vi "APC_PC_UI_Main.vi"() -> ()   [LabVIEW 2020]
uses:
  controls/APC_ControlSettings.ctl
  controls/APC_PIDcontrolSettings.ctl
  controls/APC_SavingFile.ctl
  controls/APC_ErrorCluster.ctl
panel:
  in  "Tab Control 2":enum32{"Main view", "Aux", "Test"}(tab)
  out "PYTHON \n(effective)":bool
  in  "Python in \ncommand":bool
  out "Cylinder pressure state":u32[][](array[colorbox])
  out "CA50 [CADATDC]":dbl format="%#.2f"
  in  "CA50 ref [CADBTDC]":dbl
  out "SA [CADBTDC]":dbl format="%#_2f"
  in  "Listbox":i32(listbox)
  in  "Override system view references":bool=TRUE
  out "NG flow [kg/h]":dbl format="%#.5f"
  in  "Cycles":u16=1 min=1 max=1000
  out "Saving info":string
  in  "Transfer CRIO9056":bool
  in  "Transfer CRIO9049":bool
  in  "Test notes auto erase":string="(auto-erased note)\n"
  in  "Pre-trigger":bool
  in  "Record Button":bool
  in  "Test code":string
  in  "Test ID":u32=1
  in  "Test notes":string
  in  "CO2ref":dbl
  in  "O2ref":dbl
  in  "Pref":dbl
  out "CO2 [%]":dbl format="%#.2f"
  in  "Force motoring":bool
  in  "Force idling":bool
  out "Max p [bar]":dbl[](array[numeric]) format="%#.2g"
  out "IMEP s":dbl[](array[numeric]) format="%#.2f"
  out "IMEP [bar]":dbl[](array[numeric]) format="%#.2f"
  in  "l ref":dbl format="%#.4f"
  out "l":dbl format="%#_2f"
  in  "NG flow ref":dbl format="%#.2f"
  in  "PFI enable switch":bool=TRUE
  in  "DI duration [ms]":dbl=1.0
  in  "DI advance [CADBTDC]":dbl=160.0
  in  "DI enable switch":bool=TRUE
  in  "Spark Advance [CADBTDC]":dbl
  in  "IGN enable switch":bool=TRUE
  in  "Speed setting selector":bool
  in  "Low speed setting":dbl=900.0
  in  "High speed setting":dbl=1800.0
  in  "EMERGENCY STOP":bool
  out "Warning":bool
  in  "Clear warning":bool
  out "n [rpm]":dbl
  out "Gauge":dbl(knob)=1148.34130859375 scale=0.0..2000.0
  out "Stand-by":bool
  out "Motoring":bool
  out "Firing":bool
  out "Idling":bool
  out "Emergency":bool
  out "System pressure [bar]":dbl format="%#.2f"
  out "NOx [ppm]":dbl format="%#.1f"
  out "O2 [%]":dbl format="%#.2f"
  out "Waveform Graph":dbl[][](graph)
  in  "PFI control selector":enum32{"PFI NG flow", "CL PFI  lambda"}(radio)
  in  "CL SA CA50":bool
  in  "knock limiter":bool
  out "Texh":bool
  out "control system":bool
  out "NG feed":bool
  out "NG control":bool
  out "membrane control":bool
  out "dyno control":bool
  out "Intake vent":bool
  out "NOx contamination":bool
  out "Ar feed":bool
  out "O2 feed":bool
  out "oil pressure":bool
  out "engine cooling":bool
  out "pexh":bool
  out "oil temperature":bool
  out "exhaust vent":bool
  out "cross vent":bool
  out "O2 control":bool
  out "system pressure":bool
  out "System error lookup":u32[][](array[colorbox])
  in  "Requested mode":i8(slide) scale=-1.0..3.0
  out "9056_PCnotResponding":bool
  out "9056_9049notResponding":bool
  out "9056_MTRnotResponding":bool
  out "Iteration Count":i32
  out "SystemState":dbl
  in  "ETP resync":bool
  in  "toggle \nTDC":bool
  in  "Activate\ncylinder":bool[](array[boolean])=[TRUE, TRUE, TRUE, TRUE, TRUE, TRUE]
  out "Emergency Stop Boolean":bool
  out "After 1st box":i8
  out "After 2nd box":i8
  out "After 3rd box":i8
  out "After 4th box":i8
  # "Raster 1"
  # "Raster 2"
  # "Raster 3"
  # "Raster 4"
  # "Raster 5"
  # "monarch APC v0.1"
  # "late comb"
  # "cyclic var"
  # "misfire 1"
  # "misfire 2"
  # "misfire 3"
  # "knock"
  # "Pmax"
  # "Knock limiter disabled"
  # "CA50 Control disabled"
  # "MC lambda control disabled"
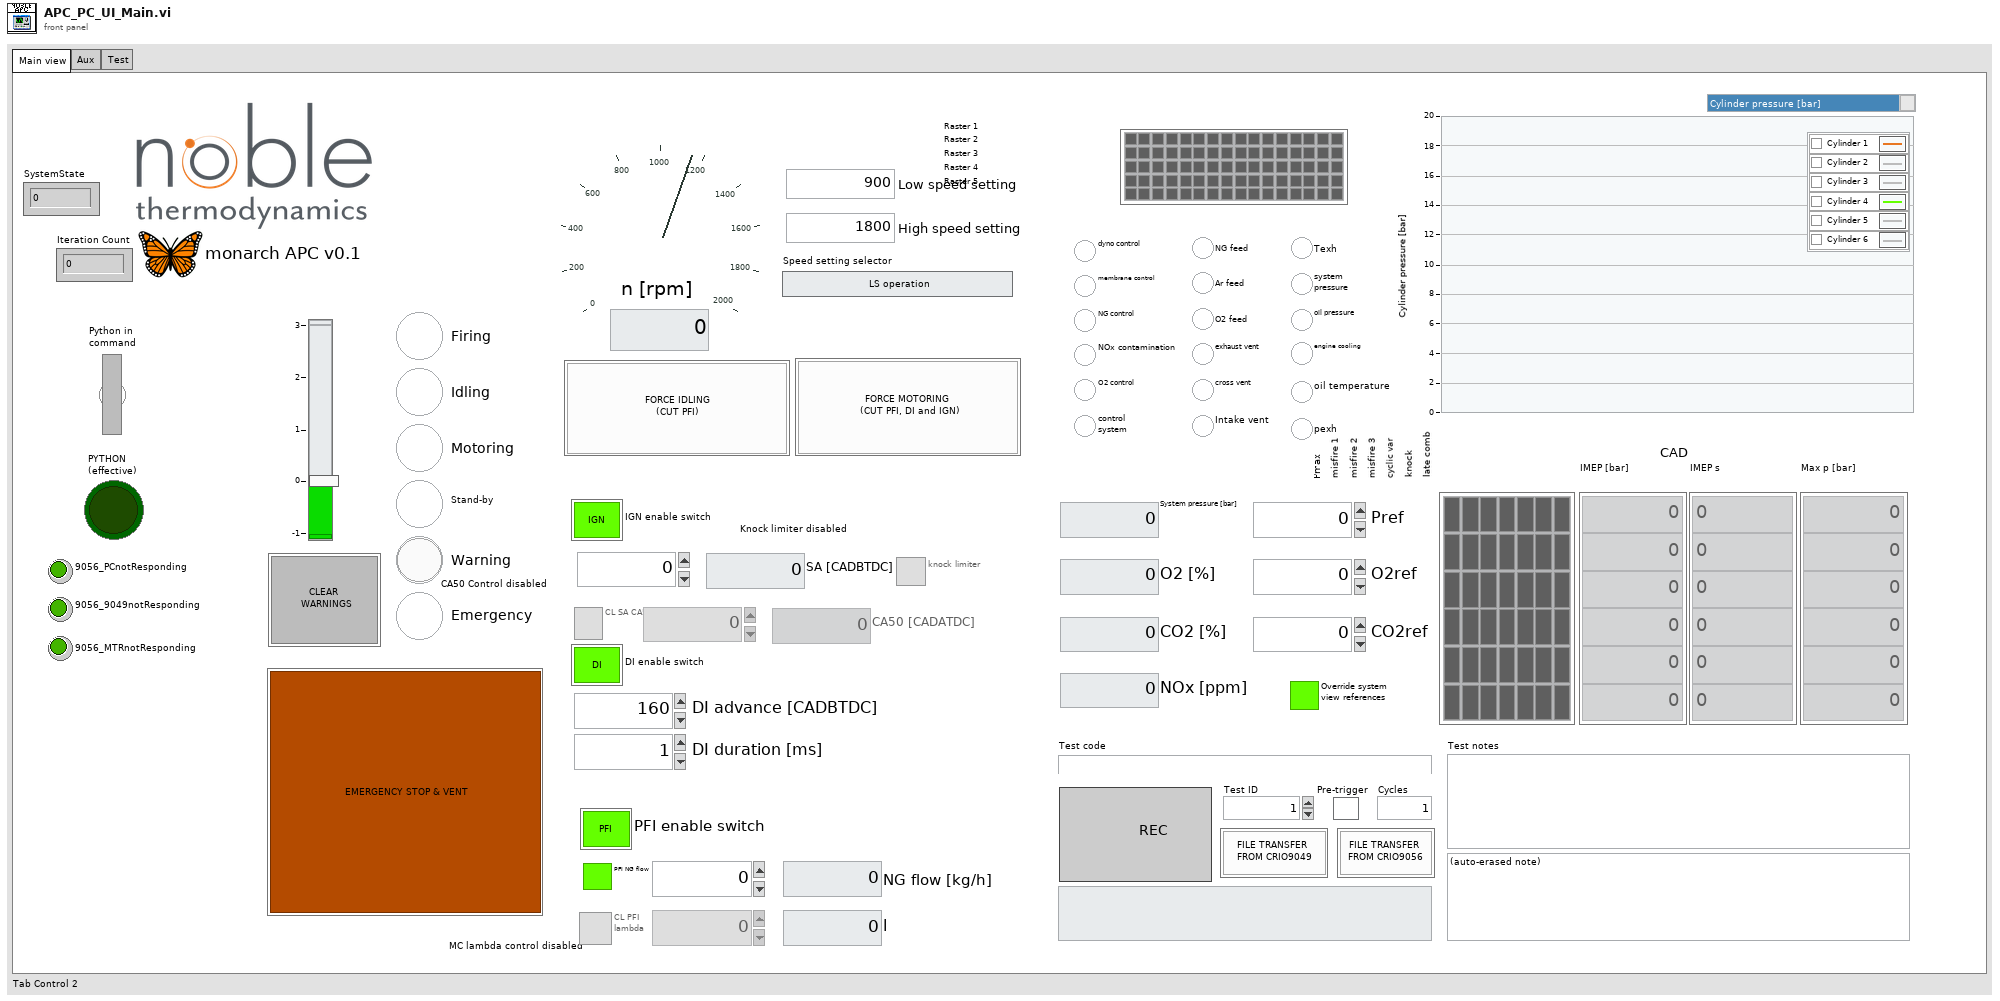
[diagram p1: front panel]
types:
  T1 = enum8{"Enabled", "Disabled", "Disabled and Grayed Out"}
  T2 = typedef "APC_ControlSettings.ctl" = cluster{"Spark advance [CADBTDC]":dbl, "Pref":dbl, "O2ref":dbl, "DI advance [CADBTDC]":dbl, "DI duration [ms] ":dbl, "CO2ref":dbl, "PFI duration [ms]":dbl, "IMEP ref":dbl, "Speed ref":dbl, "IGN enable":bool, "DI enable":bool, "CL PFI\n lambda":bool, "CL PFI\nIMEP":bool, "Activate\ncylinder":bool[], "Force idling":bool, "Force motoring":bool, "ETP resync":bool, "Requested mode":i8, "Clear Sync Errors":bool, "toggle TDC":bool, "l ref":dbl, "PID control references":T3, "CA50setpoint [CADATDC]":dbl, "CA50 control":bool, "Knock control":bool, "CLEAR EMERGENCY STOP":bool, "EMERGENCY STOP":bool}
  T3 = typedef "APC_PIDcontrolSettings.ctl" = cluster{"NG":bool, "Ar":bool, "O2":bool, "Intake vent":bool, "Cross vent":bool, "Exhaust vent":bool, "NG control mode":u8, "NG-FC-001-REF":dbl, "WF-OA-002-REF":dbl, "IMEP-REF":dbl, "Nm-REF":dbl, "Ar control mode":u8, "AR-PC-002-REF":dbl, "WF-PT-004-REF":dbl, "O2 control mode":u8, "O2-FC-001-REF":dbl, "WF-OA-001-REF":dbl, "Tcoolant control  mode":u8, "EC-FC-001-REF":dbl, "EC-TT-001-REF":dbl, "Texh control mode":u8, "SW-FC-004-REF":dbl, "SW-FT-002-REF":dbl, "WF-TT-004-REF":dbl, "Toil control mode":u8, "SW-FC-009-REF":dbl, "SW-FT-004-REF":dbl, "EO-TT-001-REF":dbl, "AIC201_CO2_ConcTarget":dbl, "O2_FF_NG":bool, "Dyno control mode":u8, "Membrane control mode":u8, "AR-FT-001-REF":dbl, "MTR modbus floats":sgl[], "MTR modbus u16":u16[], "MTR HB":bool, "PC_HB":bool, "EMERGENCY STOP":bool}
  T4 = typedef "APC_ErrorCluster.ctl" = cluster{"AI and system state":u32[][], "Cylinder pressure state":u32[][], "EMERGENCY STOP":bool}
  T5 = typedef "APC_VisualizationCluster_v2.ctl" = cluster{"AR-FT-001":dbl, "AR-PT-001":dbl, "AR-TT-001":dbl, "AT103_CO2Conc":dbl, "AT201_CO2Conc":dbl, "C101_CompSpeed_rpm":dbl, "CO2 [%]":dbl, "EC-FC-001":dbl, "EC-TT-001":dbl, "EC-TT-002":dbl, "PC-TT-001":dbl, "PC-TT-002":dbl, "PC-TT-003":dbl, "PC-TT-004":dbl, "PC-TT-005":dbl, "PC-TT-006":dbl, "EO-PT-001":dbl, "EO-TT-001":dbl, "EO-TT-002":dbl, "FT301_Flow_kgh":dbl, "FV301_VlvPos_pc_fb":dbl, "IMEPn1":dbl, "IMEPn2":dbl, "IMEPn3":dbl, "IMEPn4":dbl, "IMEPn5":dbl, "IMEPn6":dbl, "IMEPstd1":dbl, "IMEPstd2":dbl, "IMEPstd3":dbl, "IMEPstd4":dbl, "IMEPstd5":dbl, "IMEPstd6":dbl, "NG-FC-001":dbl, "NG-FT-001":dbl, "NG-PT-001":dbl, "NG-TT-001":dbl, "NGDI-FT-001":dbl, "NGDI-PT-001":dbl, "NGDI-TT-001":dbl, "WF-OA-002-NOx":dbl, "TORQUE":dbl, "WF-OA-002-O2corr":dbl, "O2-FC-001":dbl, "O2-PT-001":dbl, "O2-TT-001":dbl, "PT103_Pressure_kPa":dbl, "PT104_Pressure_kPa":dbl, "PT106_Pressure_kPa":dbl, "PT300_Pressure_kPa":dbl, "PV103_VlvPos_pc_fb":dbl, "PV300_VlvPos_pc_fb":dbl, "MaxPcyl1":dbl, "MaxPcyl2":dbl, "MaxPcyl3":dbl, "MaxPcyl4":dbl, "MaxPcyl5":dbl, "MaxPcyl6":dbl, "SW-FC-004":dbl, "SW-FC-009":dbl, "SW-FT-001":dbl, "SW-FT-002":dbl, "SW-FT-003":dbl, "SW-FT-004":dbl, "SW-TT-001":dbl, "SW-TT-002":dbl, "SW-TT-003":dbl, "SW-TT-004":dbl, "SW-TT-005":dbl, "SW-TT-006":dbl, "SW-TT-007":dbl, "SW-TT-008":dbl, "WF-OA-001":dbl, "WF-OA-002":dbl, "WF-PT-001":dbl, "WF-PT-004":dbl, "WF-PT-005avg":dbl, "WF-PT-014":dbl, "WF-PT-015":dbl, "WF-PT-016":dbl, "WF-TT-001":dbl, "WF-TT-002":dbl, "WF-TT-003":dbl, "WF-TT-004":dbl, "WF-TT-007":dbl, "EngineSpeed_rpm":dbl, "SystemState":dbl, "CylPresWarnings":dbl, "CylPresErrors":dbl, "MAPO1":dbl, "MAPO2":dbl, "MAPO3":dbl, "MAPO4":dbl, "MAPO5":dbl, "MAPO6":dbl, "CA50_1":dbl, "CA50_2":dbl, "CA50_3":dbl, "CA50_4":dbl, "CA50_5":dbl, "CA50_6":dbl, "SparkTiming":dbl, "SW-TT-009":dbl, "NG-FV-001":dbl, "O2-PV-004":dbl, "AR-PV-004":dbl, "WF-FC-001":dbl, "WF-FC-002":dbl, "WF-FC-003":dbl, "WF-PT-012avg":dbl}
  T6 = typedef "APC_SavingFile.ctl" = cluster{"TEST CODE":string, "ID":u32, "FLUSH and SAVE BUFFER":bool, "REC BUFFER":bool, "Test Notes":string, "Cycles":u16}
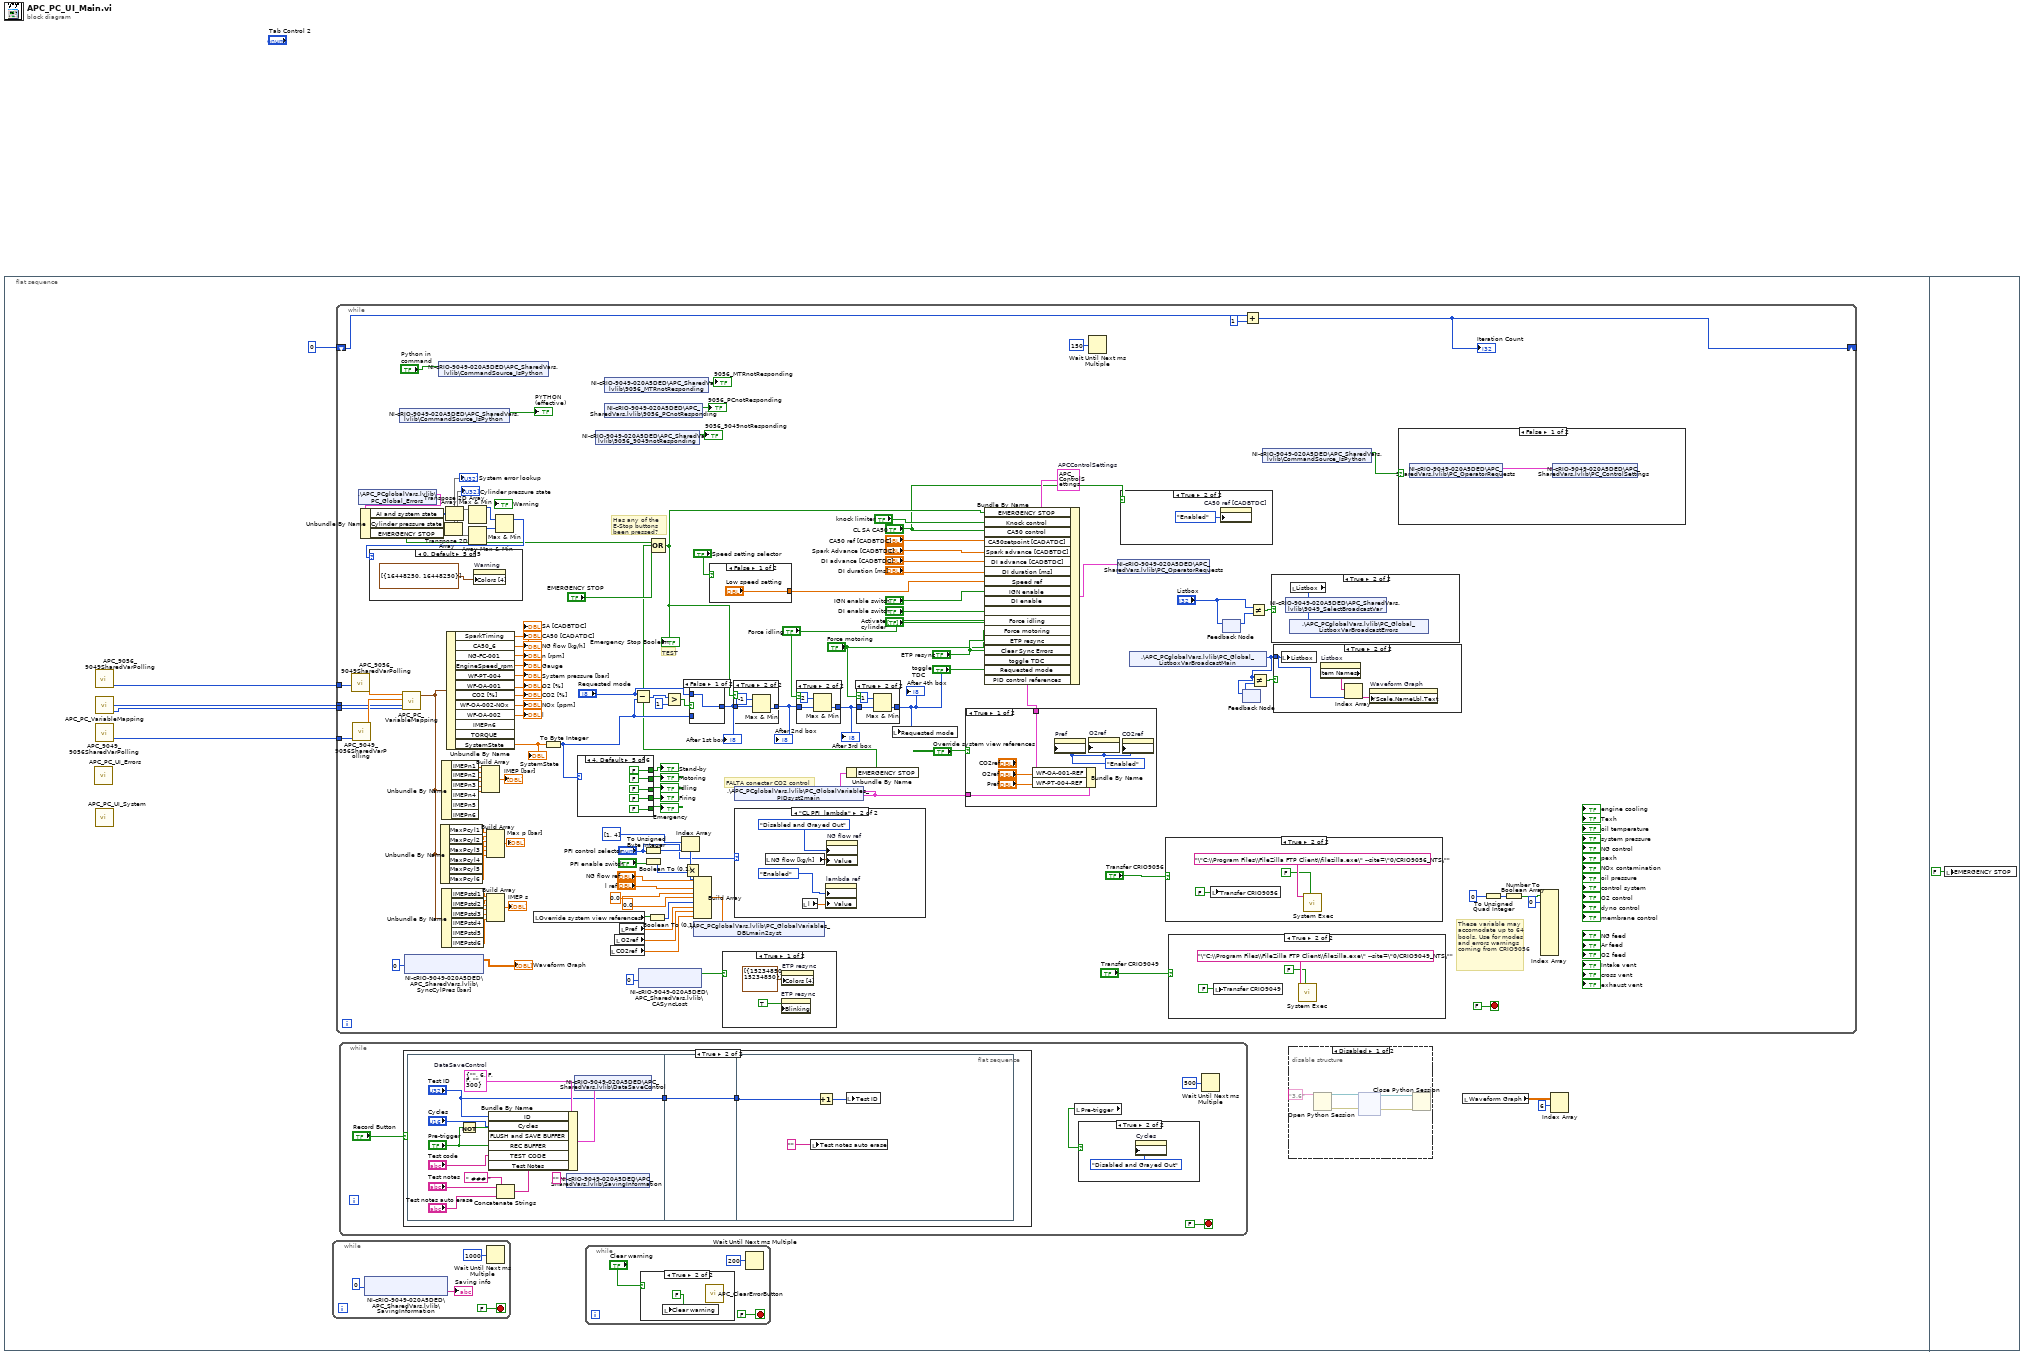
[diagram p0: block diagram]
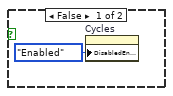
[diagram p3: hidden frame]
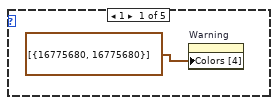
[diagram p7: hidden frame]
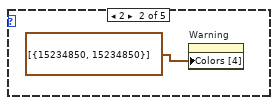
[diagram p8: hidden frame]
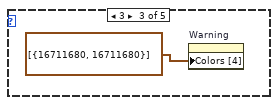
[diagram p9: hidden frame]
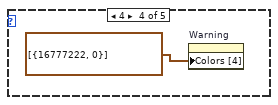
[diagram p10: hidden frame]
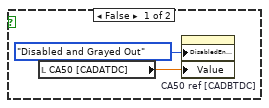
[diagram p11: hidden frame]
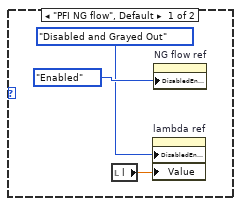
[diagram p12: hidden frame]
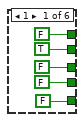
[diagram p16: hidden frame]
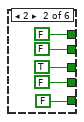
[diagram p17: hidden frame]
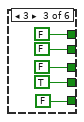
[diagram p18: hidden frame]
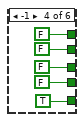
[diagram p19: hidden frame]
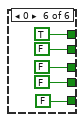
[diagram p20: hidden frame]
diagram:
  n1 = flat-sequence {
    frame #0 {
      n2 = call "APC_PC_UI_Errors.vi"() -> ()  [unwired: 12 in]
      n3 = call "APC_9056_9049SharedVarPolling.vi"() -> ("Number of signals (out)"=w5:i32)  [unwired: 1 in, 1 out]
      n4 = call "APC_PC_UI_System.vi"() -> ()  [unwired: 12 in]
      n5 = call "APC_PC_VariableMapping.vi"() -> ("Index 9056"=w6:i32[], "Index 9049"=w7:i32[])  [unwired: 4 in, 1 out]
      n6 = call "APC_9049_9056SharedVarPolling.vi"() -> ("Number of signals (out)"=w4:i32)  [unwired: 1 in, 3 out]
      n7 = while {
        stop <- FALSE stop-if-true
        n8 = shared-variable "NI-cRIO-9049-020A5DED\\APC_SharedVars.lvlib\\SavingInformation"(0 ("ms timeout (0)")) -> (→"Saving info":string)  [unwired: 1 in, 2 out]
        n9 = Wait Until Next ms Multiple(millisecond multiple=u32 1000) -> ()  [unwired: 1 out]
      }
      n10 = while {
        tunnel: w7 -> [w163]
        tunnel: w6 -> [w162]
        tunnel: w5 -> [w161]
        tunnel: w4 -> [w160]
        shift-right: [w53] -> _
        shift-left: 0 -> [w55]
        stop <- FALSE stop-if-true
        w157 = T2 {"Spark advance [CADBTDC]"=0.0, "Pref"=0.0, "O2ref"=0.0, "DI advance [CADBTDC]"=0.0, "DI duration [ms] "=0.0, "CO2ref"=0.0, "PFI duration [ms]"=0.0, "IMEP ref"=0.0, "Speed ref"=1800.0, "IGN enable"=TRUE, "DI enable"=TRUE, "CL PFI\n lambda"=FALSE, "CL PFI\nIMEP"=FALSE, "Activate\ncylinder"=[FALSE, FALSE, FALSE, FALSE, FALSE, FALSE], "Force idling"=FALSE, "Force motoring"=FALSE, "ETP resync"=FALSE, "Requested mode"=0, "Clear Sync Errors"=FALSE, "toggle TDC"=FALSE, "l ref"=0.0, "PID control references"={"NG"=FALSE, "Ar"=FALSE, "O2"=FALSE, "Intake vent"=FALSE, "Cross vent"=FALSE, "Exhaust vent"=FALSE, "NG control mode"=0, "NG-FC-001-REF"=0.0, "WF-OA-002-REF"=0.0, "IMEP-REF"=0.0, "Nm-REF"=0.0, "Ar control mode"=0, "AR-PC-002-REF"=0.0, "WF-PT-004-REF"=0.0, "O2 control mode"=0, "O2-FC-001-REF"=0.0, "WF-OA-001-REF"=0.0, "Tcoolant control  mode"=0, "EC-FC-001-REF"=0.0, "EC-TT-001-REF"=0.0, "Texh control mode"=0, "SW-FC-004-REF"=0.0, "SW-FT-002-REF"=0.0, "WF-TT-004-REF"=0.0, "Toil control mode"=0, "SW-FC-009-REF"=0.0, "SW-FT-004-REF"=0.0, "EO-TT-001-REF"=0.0, "AIC201_CO2_ConcTarget"=0.0, "O2_FF_NG"=FALSE, "Dyno control mode"=0, "Membrane control mode"=0, "AR-FT-001-REF"=0.0, "MTR modbus floats"=[0.0, 0.0, 0.0, 0.0, 0.0, 0.0, 0.0, 0.0, 0.0, 0.0, 0.0, 0.0, 0.0, 0.0, 0.0, 0.0, 0.0, 0.0, 0.0], "MTR modbus u16"=[0, 0, 0, 0, 0, 0, 0], "MTR HB"=FALSE, "PC_HB"=FALSE, "EMERGENCY STOP"=FALSE}, "CA50setpoint [CADATDC]"=0.0, "CA50 control"=TRUE, "Knock control"=FALSE, "CLEAR EMERGENCY STOP"=FALSE, "EMERGENCY STOP"=FALSE}  # APCControlSettings
        # "TEST"
        # "Has any of the E-Stop buttons been pressed?"
        # "These variable may accomodate up to 64 bools. Use for modes and errors warnings coming from CRIO9056"
        # "FALTA conectar CO2 control"
        n11 = call "APC_9056_9049SharedVarPolling.vi"("Number of signals"=w161) -> ("9049_CycleAveragedVariables"=w165:dbl[])  [unwired: 1 out]
        n12 = call "APC_9049_9056SharedVarPolling.vi"("Number of signals"=w160) -> ("9056 IO"=w164:dbl[])  [unwired: 3 out]
        n13 = shared-variable ".\\APC_PCglobalVars.lvlib\\PC_Global_Errors"() -> (w74:T4)  [unwired: 1 in, 1 out]
        n14 = Unbundle By Name(w74) -> ("AI and system state"=w72:u32[][], "Cylinder pressure state"=w73:u32[][], "EMERGENCY STOP"=w66:bool)
        n15 = shared-variable "NI-cRIO-9049-020A5DED\\APC_SharedVars.lvlib\\CommandSource_IsPython"() -> (→"PYTHON \n(effective)":bool)  [unwired: 1 in, 1 out]
        n16 = call "APC_PC_VariableMapping.vi"("Index of array for 9056"=w162, "Index of array for 9049"=w163, "9056 IO"=w164, "9049_CycleAveragedVariables"=w165) -> ("Output cluster"=w61:T5)  [unwired: 2 out]
        n17 = shared-variable "NI-cRIO-9049-020A5DED\\APC_SharedVars.lvlib\\SyncCylPres [bar]"(0 ("ms timeout (0)")) -> (→"Waveform Graph":dbl[][])  [unwired: 1 in, 2 out]
        n18 = shared-variable "NI-cRIO-9049-020A5DED\\APC_SharedVars.lvlib\\CommandSource_IsPython"("Python in \ncommand") -> ()  [unwired: 1 in, 1 out]
        n19 = Unbundle By Name(w61) -> ("MaxPcyl1"=w138:dbl, "MaxPcyl2"=w139:dbl, "MaxPcyl3"=w134:dbl, "MaxPcyl4"=w135:dbl, "MaxPcyl5"=w136:dbl, "MaxPcyl6"=w137:dbl)
        n20 = Unbundle By Name(w61) -> ("IMEPn1"=w145:dbl, "IMEPn2"=w146:dbl, "IMEPn3"=w141:dbl, "IMEPn4"=w142:dbl, "IMEPn5"=w143:dbl, "IMEPn6"=w144:dbl)
        n21 = Unbundle By Name(w61) -> ("IMEPstd1"=w131:dbl, "IMEPstd2"=w132:dbl, "IMEPstd3"=w127:dbl, "IMEPstd4"=w128:dbl, "IMEPstd5"=w129:dbl, "IMEPstd6"=w130:dbl)
        n22 = Transpose 2D Array(2D array=w73) -> (transposed array=w71:u32[][])
        "Cylinder pressure state" <- w71
        n23 = Transpose 2D Array(2D array=w72) -> (transposed array=w70:u32[][])
        "System error lookup" <- w70
        n24 = Unbundle By Name(w61) -> ("SparkTiming"=→"SA [CADBTDC]":dbl, "CA50_6"=→"CA50 [CADATDC]":dbl, "NG-FC-001"=→"NG flow [kg/h]":dbl, "EngineSpeed_rpm"=→"Gauge" →"n [rpm]":dbl, "WF-PT-004"=→"System pressure [bar]":dbl, "WF-OA-001"=→"O2 [%]":dbl, "CO2 [%]"=→"CO2 [%]":dbl, "WF-OA-002-NOx"=→"NOx [ppm]":dbl, "WF-OA-002"=→"l":dbl, "SystemState"=w91:dbl)  [unwired: 2 out]
        "SystemState" <- w91
        n25 = Array Max & Min(array=w71) -> (max value=w69:u32)  [unwired: 3 out]
        n26 = Array Max & Min(array=w70) -> (max value=w68:u32)  [unwired: 3 out]
        n27 = Build Array(w145, w146, w141, w142, w143, w144) -> (→"IMEP [bar]":dbl[])
        n28 = Build Array(w138, w139, w134, w135, w136, w137) -> (→"Max p [bar]":dbl[])
        n29 = Build Array(w131, w132, w127, w128, w129, w130) -> (→"IMEP s":dbl[])
        n30 = Max & Min(x=w69, y=w68) -> (max(x,y)=w67:u32)  [unwired: 1 out]
        n31 = case shown="0, Default" w67 {
          frame 1 {
            n32 = property on="Warning" class="Bool (strict)"("Colors [4]"=cluster{u32, u32}[] [{16775680, 16775680}]) -> ()  [unwired: 2 in, 2 out]
          }
          frame 2 {
            n33 = property on="Warning" class="Bool (strict)"("Colors [4]"=cluster{u32, u32}[] [{15234850, 15234850}]) -> ()  [unwired: 2 in, 2 out]
          }
          frame 3 {
            n34 = property on="Warning" class="Bool (strict)"("Colors [4]"=cluster{u32, u32}[] [{16711680, 16711680}]) -> ()  [unwired: 2 in, 2 out]
          }
          frame 4 {
            n35 = property on="Warning" class="Bool (strict)"("Colors [4]"=cluster{u32, u32}[] [{16777222, 0}]) -> ()  [unwired: 2 in, 2 out]
          }
          frame 0, Default {
            n36 = property on="Warning" class="Bool (strict)"("Colors [4]"=cluster{u32, u32}[] [{16448250, 16448250}]) -> ()  [unwired: 2 in, 2 out]
          }
        }
        n37 = local read "Override system view references"() -> (w105:bool)
        n38 = To Byte Integer(number=w91) -> (8bit integer=w90:i8)
        n39 = case shown="4, Default" w90 {
          tunnel: [FALSE ("Stand-by") FALSE ("Stand-by") FALSE ("Stand-by") FALSE ("Stand-by") FALSE ("Stand-by") TRUE ("Stand-by")] -> w89
          tunnel: [TRUE ("Stand-by") FALSE ("Stand-by") FALSE ("Stand-by") FALSE ("Stand-by") FALSE ("Stand-by") FALSE ("Stand-by")] -> w87
          tunnel: [FALSE ("Stand-by") FALSE ("Stand-by") FALSE ("Stand-by") TRUE ("Stand-by") FALSE ("Stand-by") FALSE ("Stand-by")] -> w88
          tunnel: [FALSE ("Stand-by") TRUE ("Stand-by") FALSE ("Stand-by") FALSE ("Stand-by") FALSE ("Stand-by") FALSE ("Stand-by")] -> w86
          tunnel: [FALSE ("Stand-by") FALSE ("Stand-by") TRUE ("Stand-by") FALSE ("Stand-by") FALSE ("Stand-by") FALSE ("Stand-by")] -> w85
          frame 1 {
          }
          frame 2 {
          }
          frame 3 {
          }
          frame -1 {
          }
          frame 4, Default {
          }
          frame 0 {
          }
        }
        "Stand-by" <- w89
        "Motoring" <- w87
        "Firing" <- w85
        "Idling" <- w86
        "Emergency" <- w88
        n40 = shared-variable "NI-cRIO-9049-020A5DED\\APC_SharedVars.lvlib\\9056_9049notResponding"() -> (→"9056_9049notResponding":bool)  [unwired: 1 in, 1 out]
        n41 = shared-variable "NI-cRIO-9049-020A5DED\\APC_SharedVars.lvlib\\9056_MTRnotResponding"() -> (→"9056_MTRnotResponding":bool)  [unwired: 1 in, 1 out]
        n42 = shared-variable "NI-cRIO-9049-020A5DED\\APC_SharedVars.lvlib\\9056_PCnotResponding"() -> (→"9056_PCnotResponding":bool)  [unwired: 1 in, 1 out]
        n43 = local read "CO2ref"() -> (w101:dbl)
        n44 = local read "O2ref"() -> (w102:dbl)
        n45 = local read "Pref"() -> (w103:dbl)
        n46 = Subtract(x="Requested mode", y=w90) -> (x-y=w93:i8)
        n47 = shared-variable "NI-cRIO-9049-020A5DED\\APC_SharedVars.lvlib\\CASyncLost"(0 ("ms timeout (0)")) -> (w60:bool)  [unwired: 1 in, 2 out]
        n48 = Boolean To (0,1)(Boolean="PFI enable switch") -> (0, 1=w119:i16)
        n49 = To Unsigned Byte Integer(number="PFI control selector") -> (unsigned 8bit integer=w78:u8)
        n50 = Boolean To (0,1)(Boolean=w105) -> (0, 1=w104:i16)
        n51 = Greater?(x=w93, y=i8 1) -> (0:w95:bool)
        n52 = Index Array(array=i16[] [1, 4] ("x*y"), index=w78) -> (element=w77:i16)
        n53 = Multiply(x=w77, y=w119) -> (x*y=w118:i16)
        n54 = case shown="False" w95 {
          tunnel: "Requested mode" -> [w231 _]
          tunnel: [w231 w232] -> w83
          tunnel: w90 -> [_ w232]
          frame False {
          }
          frame True {
          }
        }
        "After 1st box" <- w83
        n55 = Build Array(w118, "NG flow ref", "l ref", 0.0 ("element"), 0.0 ("element"), w104, w103, w102, w101) -> (w124:dbl[])
        n56 = shared-variable ".\\APC_PCglobalVars.lvlib\\PC_GlobalVariables_DBLmain2syst"(w124) -> ()  [unwired: 1 in, 1 out]
        n57 = case shown="False" "Speed setting selector" {
          tunnel: ["Low speed setting" "High speed setting"] -> w156
          frame False {
          }
          frame True {
          }
        }
        n58 = case shown="True" w60 {
          frame True {
            n59 = property on="ETP resync" class="Bool"("Blinking"=TRUE) -> ()  [unwired: 2 in, 2 out]
            n60 = property on="ETP resync" class="Bool"("Colors [4]"=cluster{u32, u32}[] [{15234850, 15234850}]) -> ()  [unwired: 2 in, 2 out]
          }
          frame False {
            n61 = property on="ETP resync" class="Bool"("Blinking"=FALSE) -> ()  [unwired: 2 in, 2 out]
            n62 = property on="ETP resync" class="Bool"("Colors [4]"=cluster{u32, u32}[] [{13816530, 13816530}]) -> ()  [unwired: 2 in, 2 out]
          }
        }
        n63 = shared-variable ".\\APC_PCglobalVars.lvlib\\PC_GlobalVariables_PIDsyst2main"() -> (w64:T3)  [unwired: 1 in, 1 out]
        n64 = case shown="\"CL PFI  lambda\"" "PFI control selector" {
          frame "PFI NG flow", Default {
            n65 = local read "l"() -> (w184:dbl)
            n66 = property on="lambda ref" class="DigNum (strict)"("DisabledEnum"=T1."Disabled and Grayed Out" ("Disabled"), "Value"=w184) -> ()  [unwired: 2 in, 2 out]
            n67 = property on="NG flow ref" class="DigNum (strict)"("DisabledEnum"=T1."Enabled" ("Disabled")) -> ()  [unwired: 2 in, 2 out]
          }
          frame "CL PFI  lambda" {
            n68 = local read "NG flow [kg/h]"() -> (w188:dbl)
            n69 = local read "l"() -> (w187:dbl)
            n70 = property on="lambda ref" class="DigNum (strict)"("DisabledEnum"=T1."Enabled" ("Disabled"), "Value"=w187) -> ()  [unwired: 2 in, 2 out]
            n71 = property on="NG flow ref" class="DigNum (strict)"("DisabledEnum"=T1."Disabled and Grayed Out" ("Disabled"), "Value"=w188) -> ()  [unwired: 2 in, 2 out]
          }
        }
        n72 = Unbundle By Name(w64) -> ("EMERGENCY STOP"=w63:bool)
        n73 = Compound Arithmetic op=OR(w66, w63, "EMERGENCY STOP") -> (w62:bool)
        "Emergency Stop Boolean" <- w62
        n74 = case shown="True" w62 {
          tunnel: w83 -> [w197 w200]
          tunnel: [w197 w199] -> w59
          frame False {
          }
          frame True {
            n75 = Max & Min(x=i8 -1, y=w200) -> (min(x,y)=w199:i8)  [unwired: 1 out]
          }
        }
        "After 2nd box" <- w59
        n76 = case shown="True" "Force idling" {
          tunnel: w59 -> [w193 w195]
          tunnel: [w193 w196] -> w82
          frame False {
          }
          frame True {
            n77 = Max & Min(x=i8 2, y=w195) -> (min(x,y)=w196:i8)  [unwired: 1 out]
          }
        }
        "After 3rd box" <- w82
        n78 = case shown="True" "Force motoring" {
          tunnel: w82 -> [w189 w191]
          tunnel: [w189 w192] -> w79
          frame False {
          }
          frame True {
            n79 = Max & Min(x=i8 1, y=w191) -> (min(x,y)=w192:i8)  [unwired: 1 out]
          }
        }
        "After 4th box" <- w79
        n80 = local write "Requested mode"(w79) -> ()
        n81 = case shown="True" "Override system view references" {
          tunnel: w64 -> [w240 w243]
          tunnel: [w237 w243] -> w115
          frame True {
            w241 = T1."Enabled" ("Disabled")
            n82 = Bundle By Name(cluster=w240, "WF-OA-001-REF"="O2ref", "WF-PT-004-REF"="Pref") -> (w237:T3)
            n83 = property on="Pref" class="DigNum (strict)"("DisabledEnum"=w241) -> ()  [unwired: 2 in, 2 out]
            n84 = property on="O2ref" class="DigNum (strict)"("DisabledEnum"=w241) -> ()  [unwired: 2 in, 2 out]
            n85 = property on="CO2ref" class="DigNum (strict)"("DisabledEnum"=w241) -> ()  [unwired: 2 in, 2 out]
          }
          frame False {
            w246 = T1."Disabled and Grayed Out" ("Disabled")
            n86 = Unbundle By Name(w243) -> ("AIC201_CO2_ConcTarget"=w242:dbl, "WF-OA-001-REF"=w244:dbl, "WF-PT-004-REF"=w245:dbl)
            n87 = property on="Pref" class="DigNum (strict)"("DisabledEnum"=w246) -> ()  [unwired: 2 in, 2 out]
            n88 = property on="O2ref" class="DigNum (strict)"("DisabledEnum"=w246) -> ()  [unwired: 2 in, 2 out]
            n89 = local write "CO2ref"(w242) -> ()
            n90 = local write "O2ref"(w244) -> ()
            n91 = local write "Pref"(w245) -> ()
            n92 = property on="CO2ref" class="DigNum (strict)"("DisabledEnum"=w246) -> ()  [unwired: 2 in, 2 out]
          }
        }
        n93 = Bundle By Name(cluster=w157, "EMERGENCY STOP"=w62, "Knock control"="knock limiter", "CA50 control"="CL SA CA50", "CA50setpoint [CADATDC]"="CA50 ref [CADBTDC]", "Spark advance [CADBTDC]"="Spark Advance [CADBTDC]", "DI advance [CADBTDC]"="DI advance [CADBTDC]", "DI duration [ms]"="DI duration [ms]", "Speed ref"=w156, "IGN enable"="IGN enable switch", "DI enable"="DI enable switch", "Activate\ncylinder"="Activate\ncylinder", "Force idling"="Force idling", "Force motoring"="Force motoring", "ETP resync"="ETP resync", "Clear Sync Errors"="ETP resync", "toggle TDC"="toggle \nTDC", "Requested mode"=w79, "PID control references"=w115) -> (w50:T2)
        n94 = Wait Until Next ms Multiple(millisecond multiple=u32 150) -> ()  [unwired: 1 out]
        n95 = shared-variable "NI-cRIO-9049-020A5DED\\APC_SharedVars.lvlib\\PC_OperatorRequests"(w50) -> ()  [unwired: 1 in, 1 out]
        n96 = case shown="True" "CL SA CA50" {
          frame False {
            n97 = local read "CA50 [CADATDC]"() -> (w179:dbl)
            n98 = property on="CA50 ref [CADBTDC]" class="DigNum (strict)"("DisabledEnum"=T1."Disabled and Grayed Out" ("Disabled"), "Value"=w179) -> ()  [unwired: 2 in, 2 out]
          }
          frame True {
            n99 = property on="CA50 ref [CADBTDC]" class="DigNum (strict)"("DisabledEnum"=T1."Enabled" ("Disabled")) -> ()  [unwired: 2 in, 2 out]
          }
        }
        n100 = shared-variable ".\\APC_PCglobalVars.lvlib\\PC_Global_ListboxVarBroadcastMain"() -> (w109:u32)  [unwired: 1 in, 1 out]
        n101 = case shown="True" "Transfer CRIO9056" {
          frame False {
          }
          frame True {
            n102 = local write "Transfer CRIO9056"(FALSE ("Transfer files to PC")) -> ()
            n103 = call <vilib>:"System Exec.vi"("wait until completion? (T)"=FALSE, "command line"="\"C:\\Program Files\\FileZilla FTP Client\\filezilla.exe\" --site=\"0/CRIO9056_NTS\"") -> ()  [unwired: 6 in, 4 out]
          }
        }
        n104 = case shown="True" "Transfer CRIO9049" {
          frame False {
          }
          frame True {
            n105 = local write "Transfer CRIO9049"(FALSE ("Transfer files to PC")) -> ()
            n106 = call <vilib>:"System Exec.vi"("wait until completion? (T)"=FALSE, "command line"="\"C:\\Program Files\\FileZilla FTP Client\\filezilla.exe\" --site=\"0/CRIO9049_NTS\"") -> ()  [unwired: 6 in, 4 out]
          }
        }
        n107 = feedback #1() -> (w114:i32)  [unwired: 1 in]
        n108 = feedback-in #1("Listbox") -> ()
        n109 = feedback #2() -> (w110:u32)  [unwired: 1 in]
        n110 = feedback-in #2(w109) -> ()
        n111 = Add(x=w55, y=1) -> (x+y=w53:i32)
        "Iteration Count" <- w53
        n112 = Not Equal?(x="Listbox", y=w114) -> (x != y?=w113:bool)
        n113 = Not Equal?(x=w109, y=w110) -> (x != y?=w111:bool)
        n114 = shared-variable "NI-cRIO-9049-020A5DED\\APC_SharedVars.lvlib\\CommandSource_IsPython"() -> (w49:bool)  [unwired: 1 in, 1 out]
        n115 = case shown="True" w113 {
          frame False {
          }
          frame True {
            n116 = local read "Listbox"() -> (w236:i32)
            n117 = shared-variable "NI-cRIO-9049-020A5DED\\APC_SharedVars.lvlib\\9049_SelectBroadcastVar"(w236) -> ()  [unwired: 1 in, 1 out]
            n118 = shared-variable ".\\APC_PCglobalVars.lvlib\\PC_Global_ListboxVarBroadcastErrors"(w236) -> ()  [unwired: 1 in, 1 out]
          }
        }
        n119 = case shown="True" w111 {
          tunnel: w109 -> [_ w233]
          frame False {
          }
          frame True {
            n120 = local write "Listbox"(w233) -> ()
            n121 = property on="Listbox" class="LstBox (strict)"() -> ("Item Names"=w235:string[])  [unwired: 2 in, 2 out]
            n122 = Index Array(array=w235, index=w233) -> (element=w234:string)
            n123 = property on="Waveform Graph" class="WFGraph (strict)"("YScale.NameLbl.Text"=w234) -> ()  [unwired: 2 in, 2 out]
          }
        }
        n124 = case shown="False" w49 {
          frame False {
            n125 = shared-variable "NI-cRIO-9049-020A5DED\\APC_SharedVars.lvlib\\PC_OperatorRequests"() -> (w173:T2)  [unwired: 1 in, 1 out]
            n126 = shared-variable "NI-cRIO-9049-020A5DED\\APC_SharedVars.lvlib\\PC_ControlSettings"(w173) -> ()  [unwired: 1 in, 1 out]
          }
          frame True {
          }
        }
        n127 = To Unsigned Quad Integer(1:u64 0 ("number")) -> (0:w97:u64)
        n128 = Number To Boolean Array(number=w97) -> (Boolean array=w98:bool[])
        n129 = Index Array(array=w98, index #1=0 ("index")) -> ()  [unwired: 11 in, 12 out]
      }
      n130 = while {
        stop <- FALSE stop-if-true
        n131 = case shown="True" "Record Button" {
          frame False {
          }
          frame True {
            n132 = flat-sequence {
              tunnel: ["Test ID"] -> w23
              tunnel: w23 -> [w36]
              tunnel: [w36] -> w22
              tunnel: w22 -> [w38]
              frame #0 {
                w29 = T6 {"TEST CODE"="", "ID"=6, "FLUSH and SAVE BUFFER"=FALSE, "REC BUFFER"=FALSE, "Test Notes"="", "Cycles"=300}  # DataSaveControl
                n133 = Not(x="Pre-trigger") -> (.not. x?=w32:bool)
                n134 = Concatenate Strings("Test notes", " ### " ("string"), "Test notes auto erase") -> (w35:string)
                n135 = Bundle By Name(cluster=w29, "ID"="Test ID", "Cycles"="Cycles", "FLUSH and SAVE BUFFER"=w32, "REC BUFFER"="Pre-trigger", "TEST CODE"="Test code", "Test Notes"=w35) -> (w30:T6)
                n136 = shared-variable "NI-cRIO-9049-020A5DED\\APC_SharedVars.lvlib\\SavingInformation"("" ("SavingInformation")) -> ()  [unwired: 1 in, 1 out]
                n137 = shared-variable "NI-cRIO-9049-020A5DED\\APC_SharedVars.lvlib\\DataSaveControl"(w30) -> ()  [unwired: 1 in, 1 out]
              }
              frame #1 {
              }
              frame #2 {
                n138 = local write "Test notes auto erase"("" ("Test Notes")) -> ()
                n139 = Increment(x=w38) -> (x+1=w39:u32)
                n140 = local write "Test ID"(w39) -> ()
              }
            }
          }
        }
        n141 = local read "Pre-trigger"() -> (w16:bool)
        n142 = case shown="True" w16 {
          frame False {
            n143 = property on="Cycles" class="DigNum (strict)"("DisabledEnum"=T1."Enabled" ("Disabled")) -> ()  [unwired: 2 in, 2 out]
          }
          frame True {
            n144 = property on="Cycles" class="DigNum (strict)"("DisabledEnum"=T1."Disabled and Grayed Out" ("Disabled")) -> ()  [unwired: 2 in, 2 out]
          }
        }
        n145 = Wait Until Next ms Multiple(millisecond multiple=u32 500) -> ()  [unwired: 1 out]
      }
      n146 = while {
        stop <- FALSE stop-if-true
        n147 = case shown="True" "Clear warning" {
          frame False {
          }
          frame True {
            n148 = local write "Clear warning"(FALSE ("Clear warning request")) -> ()
            n149 = call "APC_ClearErrorButton.vi"() -> ()  [unwired: 1 in]
          }
        }
        n150 = Wait Until Next ms Multiple(millisecond multiple=u32 200) -> ()  [unwired: 1 out]
      }
      n151 = disable-structure shown="Disabled" {
        frame Disabled {
          n152 = Open Python Session(python version="3.6" ("Python version")) -> (session out=w41:refnum<k35>, error out=w40:errorcluster)  [unwired: 2 in]
          n153 = node(w41, w40) -> (w42:refnum<k35>, w43:errorcluster)  [unwired: 4 in, 2 out]
          n154 = Close Python Session(session in=w42, error in=w43) -> ()  [unwired: 1 out]
        }
        frame Enabled {
        }
      }
      n155 = local read "Waveform Graph"() -> (w3:dbl[][])
      n156 = Index Array(array=w3, index (row)=6) -> ()  [unwired: 1 in, 1 out]
    }
    frame #1 {
      n157 = local write "EMERGENCY STOP"(FALSE ("EMERGENCY STOP")) -> ()
    }
  }
